vi "TR_Set_List_Markings.vi"(8 "error in (no error)":errorcluster, 9 "Set mark?":enum16{"Nothing", "Done", "Wait", "Error"}(ring), 10 "Track # in":i32, 11 "MulticolumnListbox in":refnum<vi>) -> (0 "error out":errorcluster, 2 "Track # out":i32, 3 "MulticolumnListbox in out":refnum<vi>)   [LabVIEW 2018, in "Tracks Repair.lvlib"]
uses:
  Tracks Repair.lvlib
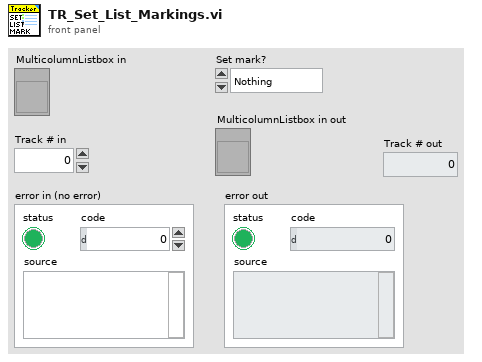
[diagram p1: front panel]
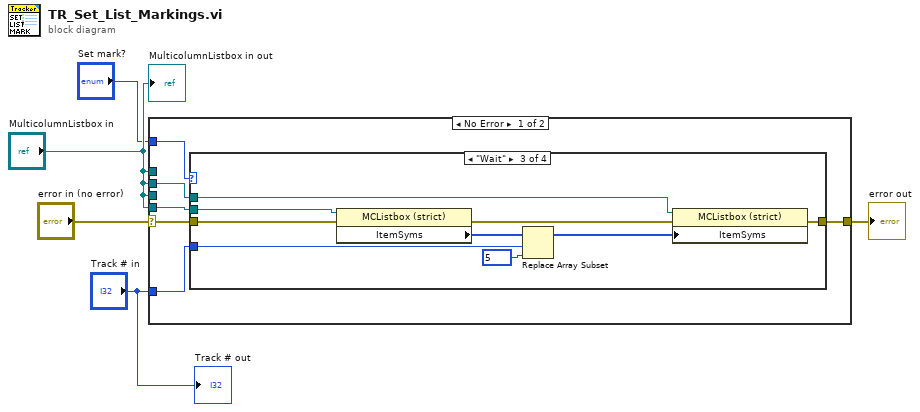
[diagram p0: block diagram]
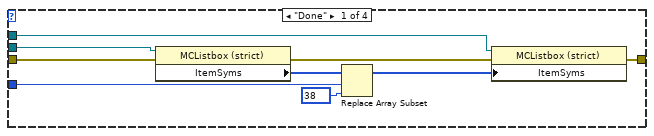
[diagram p2: hidden frame]
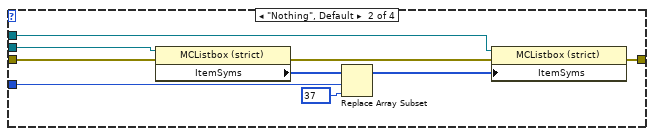
[diagram p3: hidden frame]
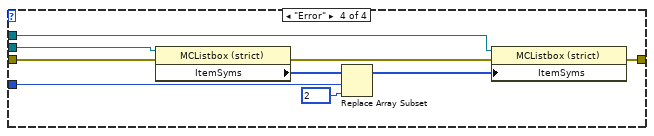
[diagram p4: hidden frame]
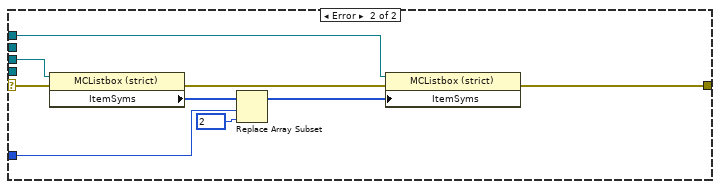
[diagram p5: hidden frame]
diagram:
  n1 = case shown="No Error" "error in (no error)" {
    selector: "error in (no error)" -> [w9 w50]
    tunnel: "Track # in" -> [w11 w55]
    tunnel: [w10 w51] -> w4
    tunnel: "MulticolumnListbox in" -> [w8 _]
    tunnel: "MulticolumnListbox in" -> [w7 _]
    tunnel: "MulticolumnListbox in" -> [_ w49]
    tunnel: "MulticolumnListbox in" -> [_ w48]
    tunnel: "Set mark?" -> [w6 _]
    frame No Error {
      n2 = case shown="\"Wait\"" w6 {
        tunnel: w11 -> [w19 w28 w37 w46]
        tunnel: [w15 w24 w33 w42] -> w10
        tunnel: w9 -> [w14 w23 w32 w41]
        tunnel: w8 -> [w13 w22 w31 w40]
        tunnel: w7 -> [w12 w21 w30 w39]
        frame "Done" {
          n3 = property on="Property Node" class="MCListbox (strict)"(reference=w13, error in=w14) -> (error out=w16:errorcluster, "ItemSyms"=w20:i32[])  [unwired: 1 out]
          n4 = Replace Array Subset(array=w20, new element=38, index=w19) -> (w18:i32[])
          n5 = property on="Property Node" class="MCListbox (strict)"(reference=w12, error in=w16, "ItemSyms"=w18) -> (error out=w15:errorcluster)  [unwired: 1 out]
        }
        frame "Nothing", Default {
          n6 = property on="Property Node" class="MCListbox (strict)"(reference=w22, error in=w23) -> (error out=w25:errorcluster, "ItemSyms"=w29:i32[])  [unwired: 1 out]
          n7 = Replace Array Subset(array=w29, new element=37, index=w28) -> (w27:i32[])
          n8 = property on="Property Node" class="MCListbox (strict)"(reference=w21, error in=w25, "ItemSyms"=w27) -> (error out=w24:errorcluster)  [unwired: 1 out]
        }
        frame "Wait" {
          n9 = property on="Property Node" class="MCListbox (strict)"(reference=w31, error in=w32) -> (error out=w34:errorcluster, "ItemSyms"=w38:i32[])  [unwired: 1 out]
          n10 = Replace Array Subset(array=w38, new element=5, index=w37) -> (w36:i32[])
          n11 = property on="Property Node" class="MCListbox (strict)"(reference=w30, error in=w34, "ItemSyms"=w36) -> (error out=w33:errorcluster)  [unwired: 1 out]
        }
        frame "Error" {
          n12 = property on="Property Node" class="MCListbox (strict)"(reference=w40, error in=w41) -> (error out=w43:errorcluster, "ItemSyms"=w47:i32[])  [unwired: 1 out]
          n13 = Replace Array Subset(array=w47, new element=2, index=w46) -> (w45:i32[])
          n14 = property on="Property Node" class="MCListbox (strict)"(reference=w39, error in=w43, "ItemSyms"=w45) -> (error out=w42:errorcluster)  [unwired: 1 out]
        }
      }
    }
    frame Error {
      n15 = property on="Property Node" class="MCListbox (strict)"(reference=w49, error in=w50) -> (error out=w52:errorcluster, "ItemSyms"=w56:i32[])  [unwired: 1 out]
      n16 = Replace Array Subset(array=w56, new element=2, index=w55) -> (w54:i32[])
      n17 = property on="Property Node" class="MCListbox (strict)"(reference=w48, error in=w52, "ItemSyms"=w54) -> (error out=w51:errorcluster)  [unwired: 1 out]
    }
  }
  "error out" <- w4
  "MulticolumnListbox in out" <- "MulticolumnListbox in"
  "Track # out" <- "Track # in"
